vi "BRig_Host__Loop_Producer__tcp_System__Data_storeFiles.vi"(0 "input_arrPath_source_wExpPrefix":path[](array[path]), 1 "input_exist_sourceAny":bool[](array[boolean]), 2 "input_exist_source":bool[](array[boolean]), 3 "input_exist_source_wExpPrefix":bool[](array[boolean]), 5 "input_arrPath_source":path[](array[path]), 7 "input_arrPath_target_wExpPrefix":path[](array[path]), 9 "input_arrPath_target":path[](array[path]), 11 "input_n":i32, 12 "input_store_wExpPrefix":bool[](array[boolean]), 13 "input_storeAny":bool[](array[boolean])) -> (4 "output_stored_wExpPrefix":bool[](array[boolean]), 8 "output_storedAny":bool[](array[boolean]))   [LabVIEW 2014]
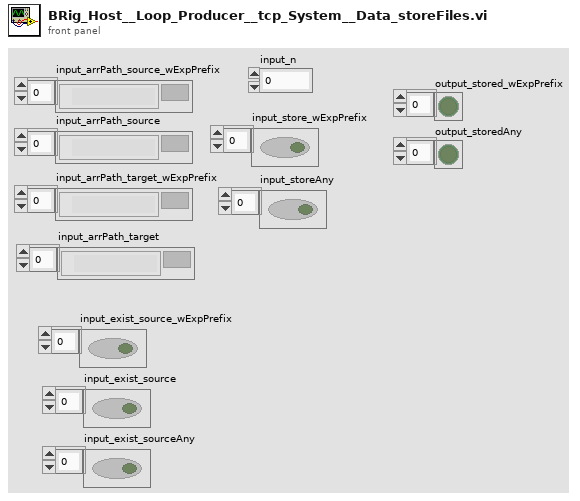
[diagram p1: front panel]
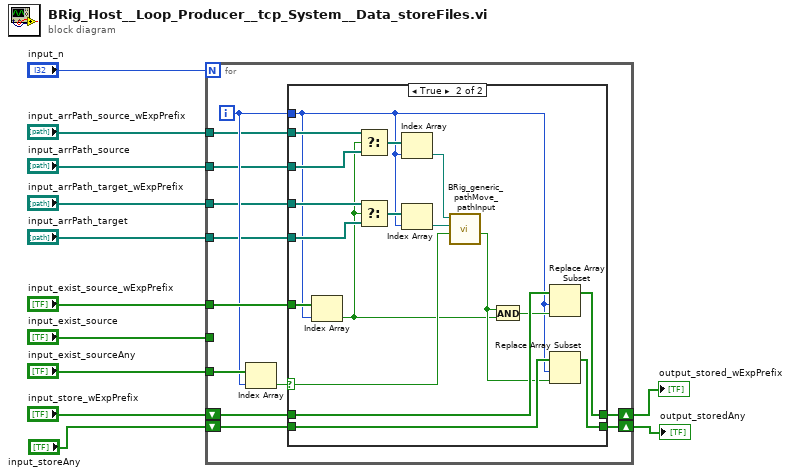
[diagram p0: block diagram]
diagram:
  n1 = for {
    N: "input_n" -> [_]
    tunnel: "input_arrPath_source" -> [w19]
    tunnel: "input_arrPath_source_wExpPrefix" -> [w20]
    tunnel: "input_arrPath_target_wExpPrefix" -> [w18]
    tunnel: "input_arrPath_target" -> [w17]
    tunnel: "input_exist_sourceAny" -> [w24]
    tunnel: "input_exist_source" -> [_]
    tunnel: "input_exist_source_wExpPrefix" -> [w22]
    shift-right: [w14] -> w3
    shift-left: "input_store_wExpPrefix" -> [w16]
    shift-right: [w13] -> w2
    shift-left: "input_storeAny" -> [w15]
    i -> [w21]
    n2 = Index Array(array=w24, index=w21) -> (element=w23:bool)
    n3 = case shown="True" w23 {
      selector: w23 -> [_ w35]
      tunnel: w22 -> [_ w44]
      tunnel: w21 -> [_ w31]
      tunnel: w20 -> [_ w43]
      tunnel: w19 -> [_ w42]
      tunnel: w18 -> [_ w41]
      tunnel: w17 -> [_ w40]
      tunnel: w16 -> [w26 w34]
      tunnel: w15 -> [w25 w32]
      tunnel: [w26 w28] -> w14
      tunnel: [w25 w29] -> w13
      frame False {
      }
      frame True {
        n4 = Index Array(array=w44, index=w31) -> (element=w27:bool)
        n5 = Select(t=w43, s=w27, f=w42) -> (s? t:f=w39:path[])
        n6 = Select(t=w41, s=w27, f=w40) -> (s? t:f=w38:path[])
        n7 = Index Array(array=w39, index=w31) -> (element=w36:path)
        n8 = Index Array(array=w38, index=w31) -> (element=w37:path)
        n9 = call "BRig_generic_pathMove_pathInput.vi"("input_Ioverwrite"=w35, "input_filePath_target"=w37, "input_filePath_source"=w36) -> ("output_Iexist"=w30:bool)  [unwired: 6 in, 2 out]
        n10 = And(x=w30, y=w27) -> (x .and. y?=w33:bool)
        n11 = Replace Array Subset(array=w34, new element=w33, index=w31) -> (w28:bool[])
        n12 = Replace Array Subset(array=w32, new element=w30, index=w31) -> (w29:bool[])
      }
    }
  }
  "output_stored_wExpPrefix" <- w3
  "output_storedAny" <- w2
